vi "UMLEditor setDiagramInfo.vi"(1 "name":string, 2 "saveDir":path, 5 "error in (no error)":errorcluster, 6 "localVariablesIn":T1 {"ObjectHotspots"."HotSpot"."y" format="%.2f"; "ObjectHotspots"."HotSpot"."x" format="%.2f"; "NodesBounds"."height" format="%.2f"; "NodesBounds"."width" format="%.2f"; "NodesBounds"."y" format="%.2f"; "NodesBounds"."x" format="%.2f"; "offset"."y" format="%.2f"; "offset"."x" format="%.2f"; "gridSize" format="%.2f"; "dragStartBounds"."height" format="%.2f"; "dragStartBounds"."width" format="%.2f"; "dragStartBounds"."y" format="%.2f"; "dragStartBounds"."x" format="%.2f"; "dragStartPoint"."y" format="%.2f"; "dragStartPoint"."x" format="%.2f"; "rubberBandStart"."y" format="%.2f"; "rubberBandStart"."x" format="%.2f"; "lastMousePoint"."y" format="%.2f"; "lastMousePoint"."x" format="%.2f"; "zoom" format="%.2f"}, 8 "action":enum16{"Name/Dir", "Unsaved", "Saved"}(ring)) -> (12 "localVariablesOut":T1 {"ObjectHotspots"."HotSpot"."y" format="%.2f"; "ObjectHotspots"."HotSpot"."x" format="%.2f"; "NodesBounds"."height" format="%.2f"; "NodesBounds"."width" format="%.2f"; "NodesBounds"."y" format="%.2f"; "NodesBounds"."x" format="%.2f"; "offset"."y" format="%.2f"; "offset"."x" format="%.2f"; "gridSize" format="%.2f"; "dragStartBounds"."height" format="%.2f"; "dragStartBounds"."width" format="%.2f"; "dragStartBounds"."y" format="%.2f"; "dragStartBounds"."x" format="%.2f"; "dragStartPoint"."y" format="%.2f"; "dragStartPoint"."x" format="%.2f"; "rubberBandStart"."y" format="%.2f"; "rubberBandStart"."x" format="%.2f"; "lastMousePoint"."y" format="%.2f"; "lastMousePoint"."x" format="%.2f"; "zoom" format="%.2f"}, 19 "error out":errorcluster)   [LabVIEW 2014]
doc: "Gets current diagram values"
uses:
  <resource>/Framework/Providers/Open_GDS/UML/UMLEditor/UMLEditor LocalVariablesType.ctl
  <resource>/Framework/Providers/Open_GDS/UML/Graphics_class/Graphics.lvclass
  <resource>/Framework/Providers/Open_GDS/UML/Grid_class/Grid.lvclass
  <resource>/Framework/Providers/Open_GDS/UML/AbstractEdge_class/AbstractEdge.lvclass
  <resource>/Framework/Providers/Open_GDS/UML/AbstractNode_class/AbstractNode.lvclass
  <resource>/Framework/Providers/Open_GDS/UML/UMLEditor/UMLEditor statesType.ctl
  <resource>/Framework/Providers/Open_GDS/UML/UMLEditor/UMLEditor tooltype.ctl
  <resource>/Framework/Providers/Open_GDS/UML/UMLEditor/UMLEditor_DiagramInfo.ctl
  <resource>/Framework/Providers/Open_GDS/UML/Graph_class/Graph.lvclass
  <resource>/Framework/Providers/Open_GDS/UML/General/Point/Point Point2D.ctl
  <resource>/Framework/Providers/Open_GDS/UML/General/Rectangle/Rectangle Rectangle2D.ctl
  <resource>/Framework/Providers/Open_GDS/UML/UMLEditor/UMLEditor ExportType.ctl
  <resource>/Framework/Providers/Open_GDS/UML/UMLEditor/UMLEditor FlattenCommandType.ctl
  <resource>/Framework/Providers/Open_GDS/UML/UMLEditor/UMLEditor ExecuteCommandType.ctl
  <resource>/Framework/Providers/Open_GDS/UML/ContextHelp/ContextHelp_EventType.ctl
  <resource>/Framework/Providers/Open_GDS/UML/UMLEditor/UMLEditor_HotSpotData.ctl
  <resource>/Framework/Providers/Open_GDS/UML/UMLEditor/UMLEditor_HotSpotType.ctl
  <resource>/Framework/Providers/Open_GDS/UML/UmlEditor_class/EventData.ctl
  <resource>/Framework/Providers/Open_GDS/UML/Graph_class/private/diagramType.ctl
  <resource>/Framework/Providers/Open_GDS/UML/UmlEditor_class/UmlEditor.lvclass
panel:
  in  "graph":refnum<class "Graph.lvclass">
  in  "unsaved":bool
  in  "diagramType":T13=enum."Class"
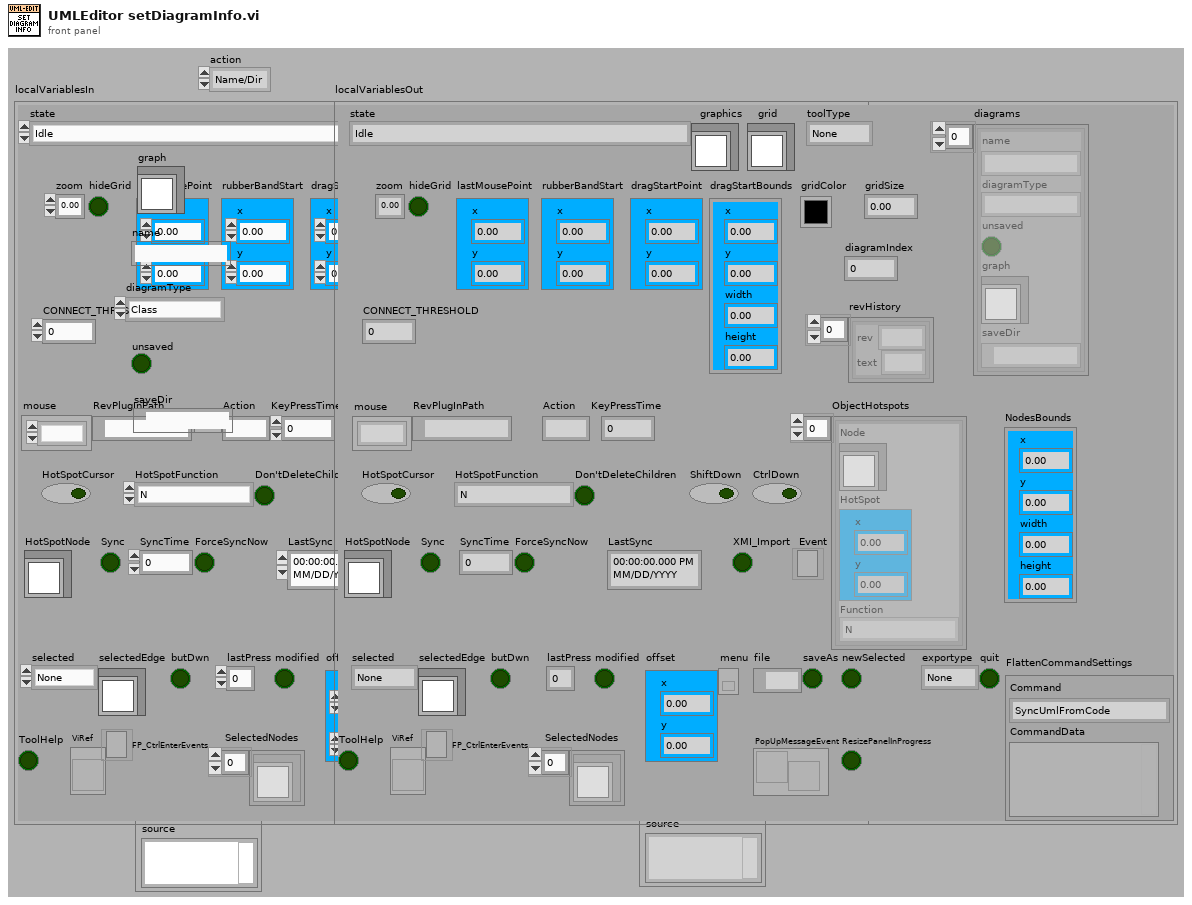
[diagram p1: front panel]
types:
  T1 = typedef "UMLEditor LocalVariablesType.ctl" = cluster{"state":T2, "graphics":refnum<class "Graphics.lvclass">, "grid":refnum<class "Grid.lvclass">, "toolType":T3, "diagramIndex":i32, "diagrams":T4[], "zoom":dbl, "hideGrid":bool, "lastMousePoint":T5, "rubberBandStart":T5, "dragStartPoint":T5, "dragStartBounds":T6, "gridColor":u32, "gridSize":dbl, "CONNECT_THRESHOLD":i32, "selected":T3, "selectedEdge":refnum<class "AbstractEdge.lvclass">, "butDwn":bool, "lastPress":u32, "modified":bool, "offset":T5, "menu":refnum<k9>, "file":path, "saveAs":bool, "newSelected":bool, "exportype":T7, "quit":bool, "revHistory":cluster{"rev":string, "text":string}[], "FlattenCommandSettings":T8, "PopUpMessageEvent":T10, "ResizePanelInProgress":bool, "NodesBounds":T6, "ToolHelp":bool, "ViRef":refnum<vi>, "FP_CtrlEnterEvents":refnum<event-registration>, "SelectedNodes":refnum<class "AbstractNode.lvclass">[], "mouse":refnum<k1>, "RevPlugInPath":path, "Action":string, "KeyPressTime":u32, "ObjectHotspots":T11[], "HotSpotCursor":bool, "HotSpotFunction":T12, "Don'tDeleteChildren":bool, "ShiftDown":bool, "CtrlDown":bool, "HotSpotNode":refnum<class "AbstractNode.lvclass">, "Sync":bool, "SyncTime":u32, "ForceSyncNow":bool, "LastSync":timestamp, "XMI_Import":bool, "Event":refnum<event-registration>}
  T2 = typedef "UMLEditor statesType.ctl" = enum16{"Idle", "CheckLicense", "revHistory", "Init", "Init2", "EditSelected", "RemoveSelected", "PaintComponent", "ChangeZoom", "ChangeGridSize", "Open", "Close", "Save", "ExportPicture", "Export", "Repaint", "Error", "Exit", "QUIT", "CreateScript", "ExecuteScript", "ClassReversedEngineering", "PlugInReverseEngineering", "StateReversedEngineering", "AutoPlace", "ExecuteCommand", "OpenClass", "SyncAll", "StraightenAssociation", "Copy", "Paste", "AddNodeFromProjectTree", "AddNodeFromProjectTree+SyncAll", "PanAndRepaint", "Init3", "CopyPaste", "ApplyDesignPattern", "AnalyseViInStateDiagram", "AutoSync"}
  T3 = typedef "UMLEditor tooltype.ctl" = enum16{"None", "Node", "Edge"}
  T4 = typedef "UMLEditor_DiagramInfo.ctl" = cluster{"name":string, "diagramType":string, "unsaved":bool, "graph":refnum<class "Graph.lvclass">, "saveDir":path}
  T5 = typedef "Point Point2D.ctl" = cluster{"x":dbl, "y":dbl}
  T6 = typedef "Rectangle Rectangle2D.ctl" = cluster{"x":dbl, "y":dbl, "width":dbl, "height":dbl}
  T7 = typedef "UMLEditor ExportType.ctl" = enum16{"None", "Printer", "png", "jpg", "roseUML"}
  T8 = typedef "UMLEditor FlattenCommandType.ctl" = cluster{"Command":T9, "CommandData":variant}
  T9 = typedef "UMLEditor ExecuteCommandType.ctl" = enum16{"SyncUmlFromCode", "SyncCodeFromUML", "OpenClass", "OpenFile", "CreateClass", "CreateVI", "OpenClassAttribute", "LocateInProject", "GraphExecute"}
  T10 = typedef "ContextHelp_EventType.ctl" = refnum<user-event>
  T11 = typedef "UMLEditor_HotSpotData.ctl" = cluster{"Node":refnum<class "AbstractNode.lvclass">, "HotSpot":T5, "Function":T12}
  T12 = typedef "UMLEditor_HotSpotType.ctl" = enum16{"N", "NE", "E", "SE", "S", "SW", "W", "NW", "Expand", "Collaps"}
  T13 = typedef "Graph.lvclass/diagramType.ctl" = enum16{"None", "Class", "Sequency", "State", "UseCase", "DQMH-Module"}
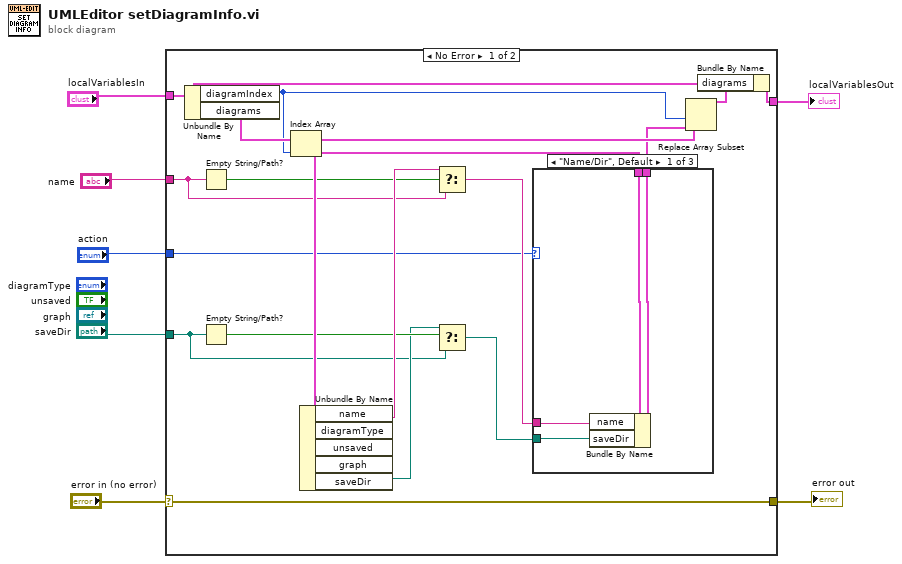
[diagram p0: block diagram]
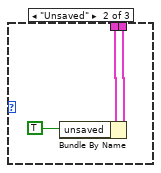
[diagram p2: hidden frame]
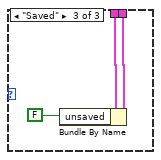
[diagram p3: hidden frame]
diagram:
  n1 = case shown="No Error" "error in (no error)" {
    selector: "error in (no error)" -> [w24 w36]
    tunnel: [w24 w36] -> w6
    tunnel: "localVariablesIn" -> [w15 w35]
    tunnel: "name" -> [w20 _]
    tunnel: [w13 w35] -> w3
    tunnel: "action" -> [w12 _]
    tunnel: "saveDir" -> [w9 _]
    frame No Error {
      n2 = Unbundle By Name(w15) -> ("diagramIndex"=w17:i32, "diagrams"=w18:T4[])
      n3 = Empty String/Path?(string/path=w20) -> (empty?=w21:bool)
      n4 = Empty String/Path?(string/path=w9) -> (empty?=w11:bool)
      n5 = Index Array(array=w18, index=w17) -> (element=w23:T4)
      n6 = Unbundle By Name(w23) -> ("name"=w22:string, "saveDir"=w10:path)  [unwired: 3 out]
      n7 = Select(t=w22, s=w21, f=w20) -> (s? t:f=w19:string)
      n8 = Select(t=w10, s=w11, f=w9) -> (s? t:f=w8:path)
      n9 = case shown="\"Name/Dir\", Default" w12 {
        tunnel: w23 -> [w28 w31 w34]
        tunnel: w19 -> [w27 _ _]
        tunnel: [w26 w30 w33] -> w16
        tunnel: w8 -> [w25 _ _]
        frame "Name/Dir", Default {
          n10 = Bundle By Name(cluster=w28, "name"=w27, "saveDir"=w25) -> (w26:T4)
        }
        frame "Unsaved" {
          n11 = Bundle By Name(cluster=w31, "unsaved"=TRUE) -> (w30:T4)
        }
        frame "Saved" {
          n12 = Bundle By Name(cluster=w34, "unsaved"=FALSE) -> (w33:T4)
        }
      }
      n13 = Replace Array Subset(array=w18, new element=w16, index=w17) -> (w14:T4[])
      n14 = Bundle By Name(cluster=w15, "diagrams"=w14) -> (w13:T1)
    }
    frame Error {
    }
  }
  "error out" <- w6
  "localVariablesOut" <- w3
